vi "Get Build Steps core.vi"(8 "error in (no error)":errorcluster, 9 "Preview?":bool, 10 "Build Configuration":string, 11 "VIPM Item in":refnum<class "VIPM Item.lvclass">) -> (0 "error out":errorcluster, 2 "Build Steps":refnum<class "Build Step.lvclass">[](array[class]))   [LabVIEW 2019, in "VIPM.lvlib" / "VIPM Item.lvclass"]
uses:
  VIPM Item.lvclass
  libs/Solution.lvlibp/Solution/Build Item/Build Step.lvclass
  VIPM Item.lvclass/VIPM Item.ctl
  Build VIPB Step/Build VIPB Step.lvclass
  C:/Users/pasca/source/repos/mgi-solution-explorer-extensions/libs/Solution.lvlibp/Solution/Build Item/Build Step.lvclass
  Apply VIPC Step/Apply VIPC Step.lvclass
  Open VIPM Step/Open VIPM Step.lvclass
  Close VIPM Step/Close VIPM Step.lvclass
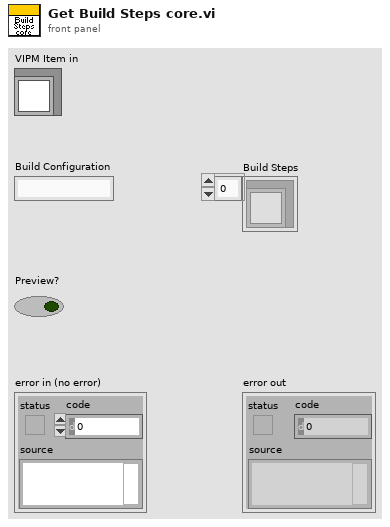
[diagram p1: front panel]
types:
  T1 = typedef "VIPM.lvlib/VIPM Item.lvclass/File Type.ctl" = enum16{"Unsupported", "VIPB", "VIPC"}
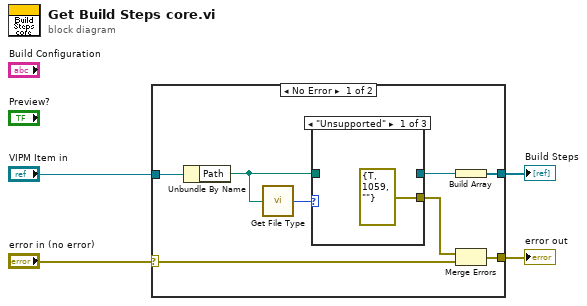
[diagram p0: block diagram]
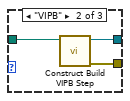
[diagram p2: hidden frame]
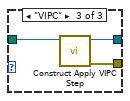
[diagram p3: hidden frame]
diagram:
  n1 = case shown="No Error" "error in (no error)" {
    selector: "error in (no error)" -> [w8 w20]
    tunnel: [w12 _] -> w4
    tunnel: [w9 w20] -> w2
    tunnel: "VIPM Item in" -> [w10 _]
    frame No Error {
      n2 = Unbundle By Name(w10) -> ("Path"=w6:path)
      n3 = call "Get File Type.vi"("Path"=w6) -> ("File Type"=w5:T1)  [unwired: 1 in]
      n4 = case shown="\"Unsupported\"" w5 {
        tunnel: [_ w16 w19] -> w11
        tunnel: [errorcluster {"status"=TRUE, "code"=1059, "source"=""} ("error constant") w15 w18] -> w7
        tunnel: w6 -> [_ w14 w17]
        frame "Unsupported" {
        }
        frame "VIPB" {
          n5 = call "Construct Build VIPB Step.vi"("Path"=w14) -> ("error out"=w15:errorcluster, "Build VIPB Step"=w16:refnum<class "Build VIPB Step.lvclass">)  [unwired: 9 in]
        }
        frame "VIPC" {
          n6 = call "Construct Apply VIPC Step.vi"("Path"=w17) -> ("error out"=w18:errorcluster, "Apply VIPC Step"=w19:refnum<class "Apply VIPC Step.lvclass">)  [unwired: 9 in]
        }
      }
      n7 = Build Array(w11) -> (w12:refnum<class "Build Step.lvclass">[])
      n8 = Merge Errors(w7, w8) -> (w9:errorcluster)
    }
    frame Error {
    }
  }
  "error out" <- w2
  "Build Steps" <- w4
